vi "ch config build array.vi"(9 "configtable":T2 {"CHS"."display" format="%b"}) -> (1 "output array":string[][](array[string]))   [LabVIEW 2011]
uses:
  contable.ctl
  CHS.ctl
  singlechtype.ctl
  gain.ctl
panel:
  out "Gain":T1
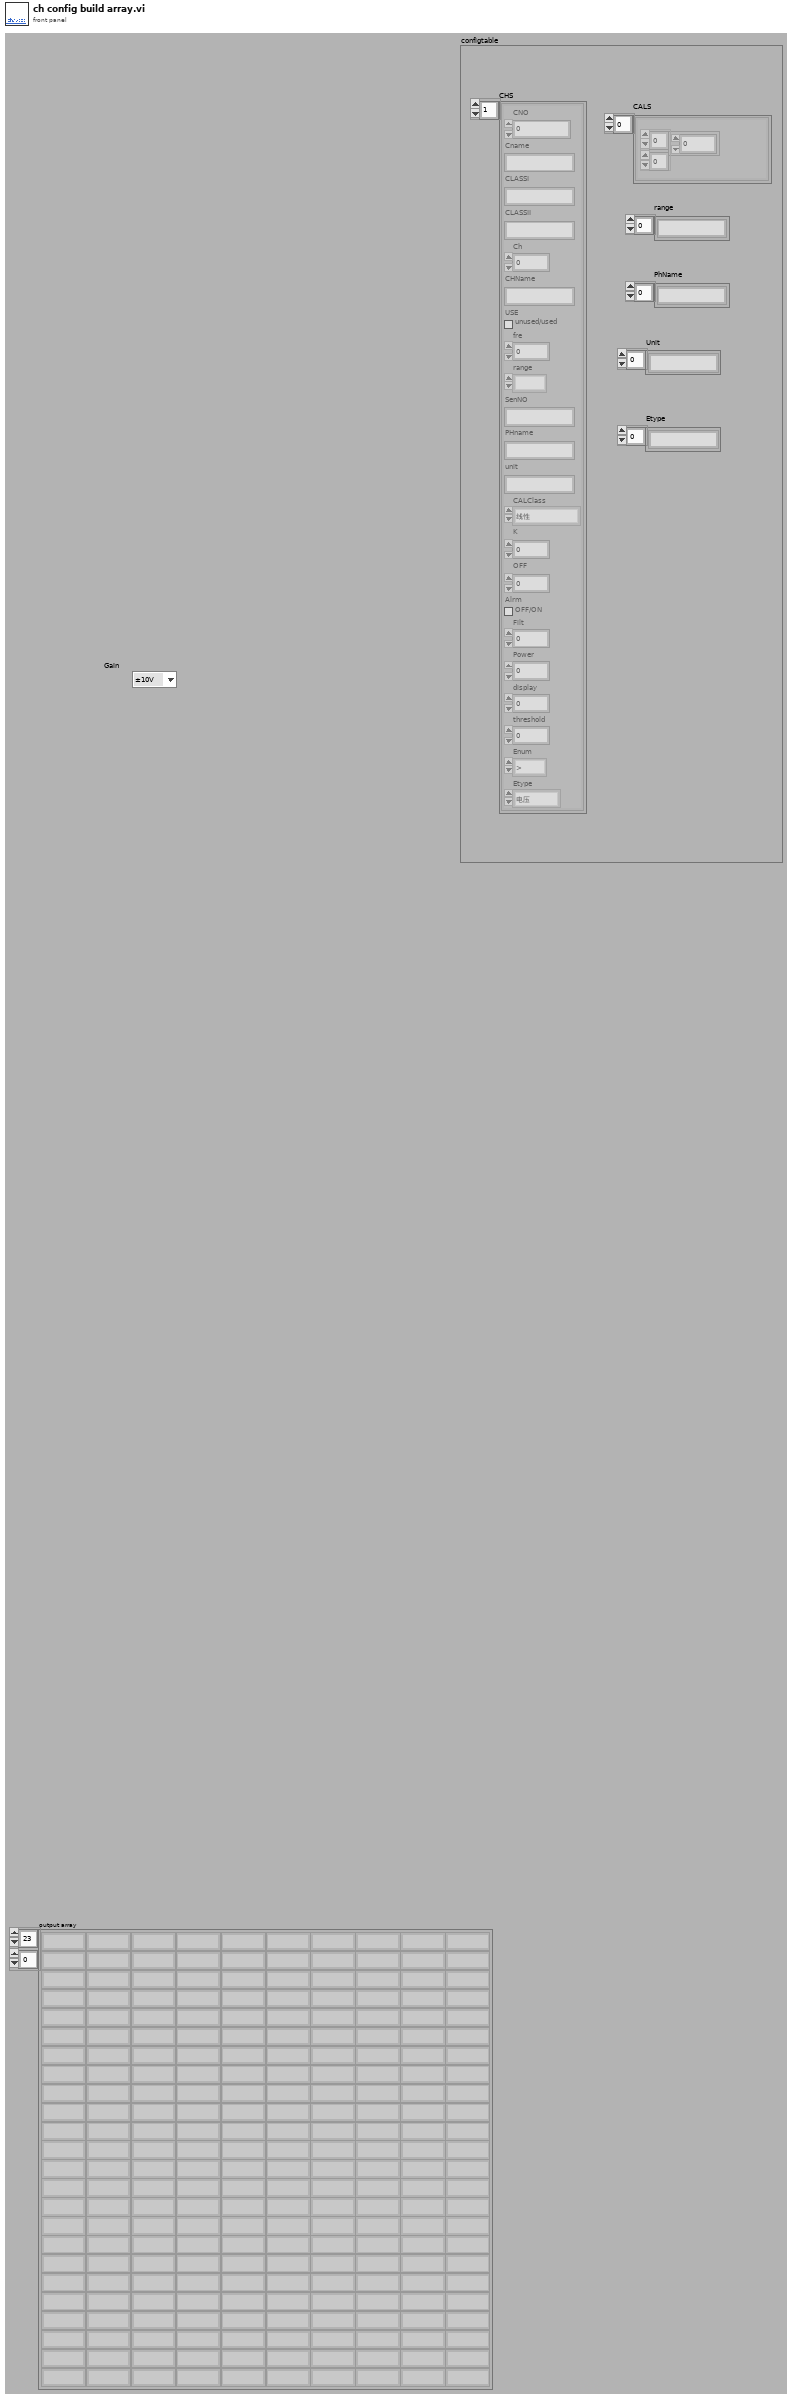
[diagram p1: front panel]
types:
  T1 = typedef "gain.ctl" = enum16{"±10V", "±5V", "±2.5V", "±1V", "±500mV", "±100mV", "10V", "5V", "2.5V", "1V", "500mV", "100mV"}
  T2 = typedef "contable.ctl" = cluster{"CHS":T3, "CALS":cluster{"Array":dbl[][]}[], "range":string[], "PhName":string[], "Unit":string[], "Etype":string[]}
  T3 = typedef "CHS.ctl" = T4[]
  T4 = typedef "singlechtype.ctl" = cluster{"CNO":u8, "Cname":string, "CLASSI":string, "CLASSII":string, "Ch":u8, "CHName":string, "USE":bool, "fre":dbl, "range":enum16{""}, "SenNO":string, "PHname":string, "unit":string, "CALClass":enum8{"线性", "查表", "公式"}, "K":dbl, "OFF":dbl, "Alrm":bool, "Filt":dbl, "Power":u8, "display":u8, "threshold ":dbl, "Enum":enum16{">", ">=", "<", "<=", "<>(在范围内）", "><（在范围外）"}, "Etype":enum16{"电压", "电流", "电阻", "热电偶K", "热电偶T"}}
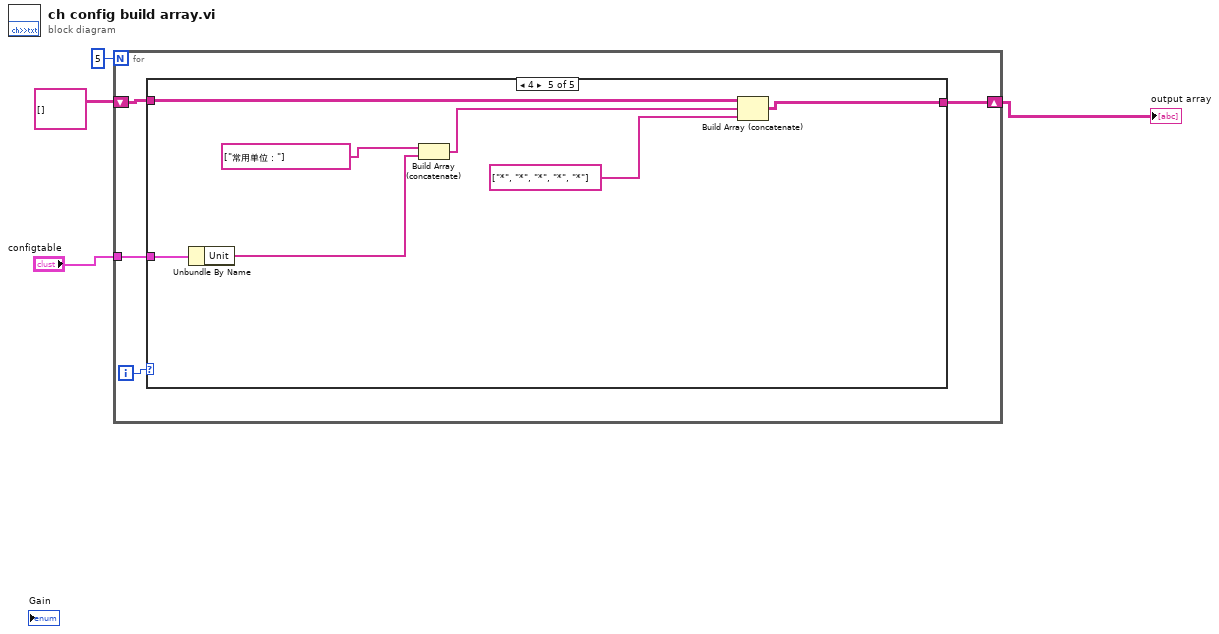
[diagram p0: block diagram]
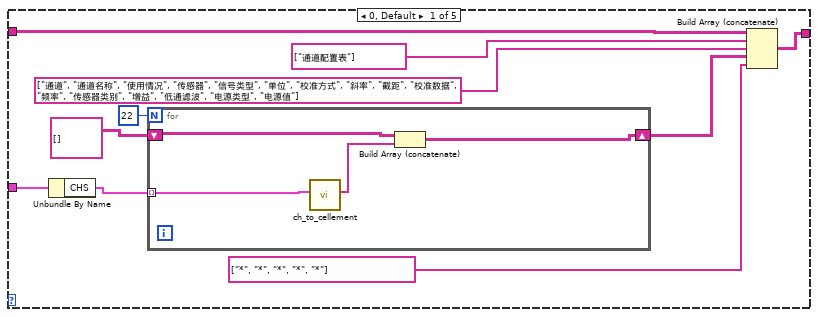
[diagram p2: hidden frame]
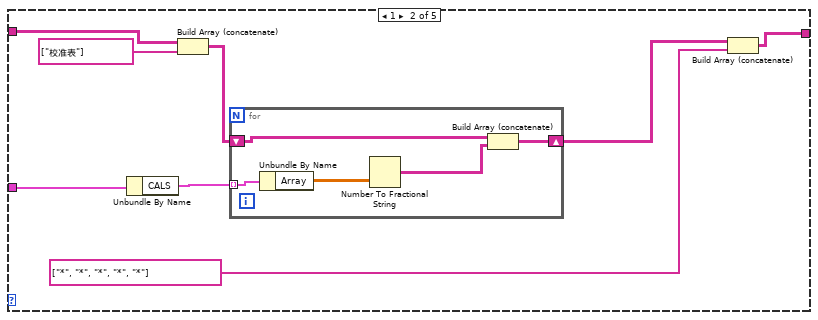
[diagram p3: hidden frame]
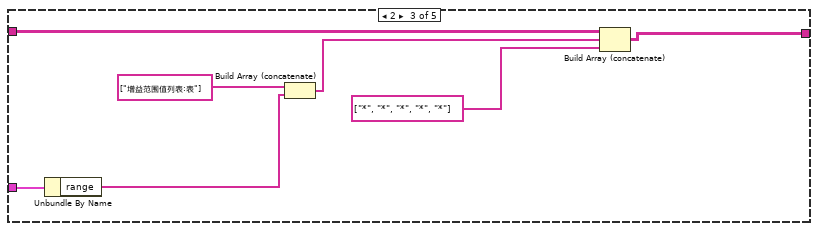
[diagram p4: hidden frame]
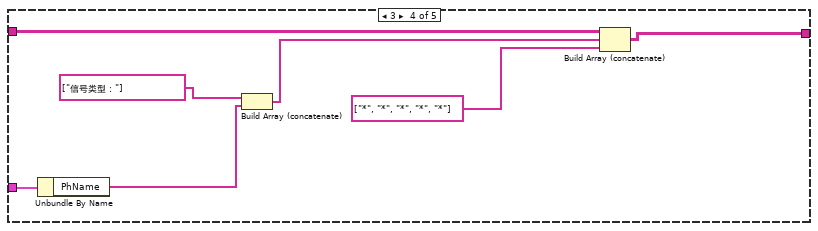
[diagram p5: hidden frame]
diagram:
  n1 = for {
    N: 5 -> [_]
    tunnel: "configtable" -> [w5]
    shift-right: [w7] -> w2
    shift-left: string[][] [] -> [w8]
    i -> [w6]
    n2 = case shown="4" w6 {
      tunnel: w8 -> [w16 w30 w42 w49 w56]
      tunnel: [w17 w24 w41 w48 w55] -> w7
      tunnel: w5 -> [w18 w29 w40 w47 w54]
      frame 0, Default {
        n3 = Unbundle By Name(w18) -> ("CHS"=w13:T3)
        n4 = for {
          N: 22 -> [_]
          tunnel: w13 -> [w22] mode=indexing
          shift-right: [w20] -> w10
          shift-left: string[][] [] -> [w21]
          n5 = call "ch_to_cellement.vi"("element"=w22) -> ("chtree cell Array"=w19:string[])  [unwired: 10 in]
          n6 = Build Array (concatenate)(w21, w19) -> (w20:string[][])
        }
        n7 = Build Array (concatenate)(w16, string[] ["通道配置表"], string[] ["通道", "通道名称", "使用情况", "传感器", "信号类型", "单位", "校准方式", "斜率", "截距", "校准数据", "频率", "传感器类别", "增益", "低通滤波", "电源类型", "电源值"], w10, string[] ["*", "*", "*", "*", "*"]) -> (w17:string[][])
      }
      frame 1 {
        n8 = Unbundle By Name(w29) -> ("CALS"=w27:cluster{"Array":dbl[][]}[])
        n9 = Build Array (concatenate)(w30, string[] ["校准表"]) -> (w26:string[][])
        n10 = for {
          tunnel: w27 -> [w35] mode=indexing
          shift-right: [w31] -> w25
          shift-left: w26 -> [w33]
          n11 = Unbundle By Name(w35) -> ("Array"=w34:dbl[][])
          n12 = Number To Fractional String(number=w34) -> (F-format string=w32:string[][])  [unwired: 3 in]
          n13 = Build Array (concatenate)(w33, w32) -> (w31:string[][])
        }
        n14 = Build Array (concatenate)(w25, string[] ["*", "*", "*", "*", "*"]) -> (w24:string[][])
      }
      frame 2 {
        n15 = Unbundle By Name(w40) -> ("range"=w37:string[])
        n16 = Build Array (concatenate)(string[] ["增益范围值列表:表"], w37) -> (w36:string[])
        n17 = Build Array (concatenate)(w42, w36, string[] ["*", "*", "*", "*", "*"] ("element")) -> (w41:string[][])
      }
      frame 3 {
        n18 = Unbundle By Name(w47) -> ("PhName"=w44:string[])
        n19 = Build Array (concatenate)(string[] ["信号类型："], w44) -> (w43:string[])
        n20 = Build Array (concatenate)(w49, w43, string[] ["*", "*", "*", "*", "*"] ("element")) -> (w48:string[][])
      }
      frame 4 {
        n21 = Unbundle By Name(w54) -> ("Unit"=w51:string[])
        n22 = Build Array (concatenate)(string[] ["常用单位："], w51) -> (w50:string[])
        n23 = Build Array (concatenate)(w56, w50, string[] ["*", "*", "*", "*", "*"] ("element")) -> (w55:string[][])
      }
    }
  }
  "output array" <- w2
